vi "optionsAcq_readError.vi"(0 "option default":u16, 2 "option return":i32, 5 "error in (no error)":errorcluster, 9 "error ignore":bool) -> (15 "status":string, 16 "option":u16, 19 "error out":errorcluster)   [LabVIEW 2010, in "OSA.lvclass"]
doc: "SubVI to a <B>Thorlabs_OSA_64</B> object.\n\n[GOOP 1.0]"
uses:
  OSA.lvclass
  OSA20X_misc.lvlib
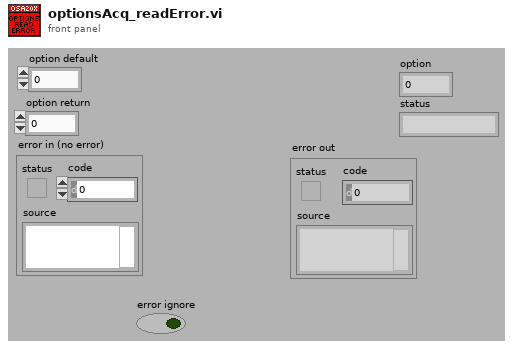
[diagram p1: front panel]
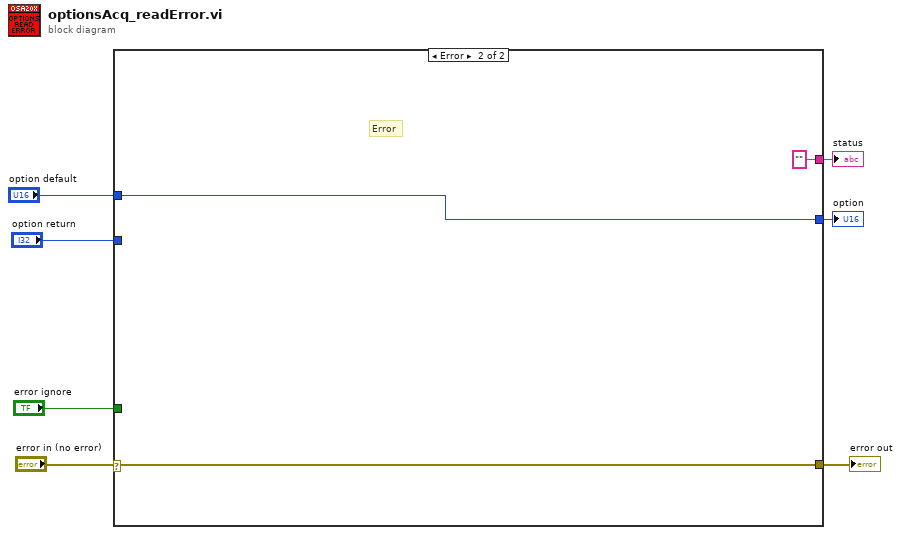
[diagram p0: block diagram]
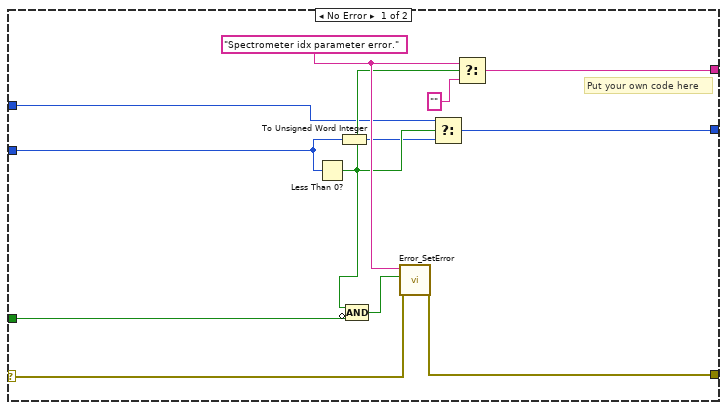
[diagram p2: hidden frame]
diagram:
  n1 = case shown="Error" "error in (no error)" {
    selector: "error in (no error)" -> [w9 w22]
    tunnel: [w8 w22] -> w7
    tunnel: "option return" -> [w14 _]
    tunnel: "option default" -> [w13 w21]
    tunnel: "error ignore" -> [w12 _]
    tunnel: [w11 w21] -> w2
    tunnel: [w10 ""] -> w1
    frame No Error {
      w18 = "Spectrometer idx parameter error." ("status")
      # "Put your own code here"
      n2 = Less Than 0?(x=w14) -> (x < 0?=w16:bool)
      n3 = To Unsigned Word Integer(number=w14) -> (unsigned 16bit integer=w15:u16)
      n4 = Compound Arithmetic op=AND(w16, invert w12) -> (w17:bool)
      n5 = call "Error_SetError.vi"("error in"=w9, "status (true)"=w17, "source(\"\")"=w18) -> ("error out"=w8:errorcluster)  [unwired: 4 in]
      n6 = Select(t=w13, s=w16, f=w15) -> (s? t:f=w11:u16)
      n7 = Select(t=w18, s=w16, f="") -> (s? t:f=w10:string)
    }
    frame Error {
      # "Error"
    }
  }
  "error out" <- w7
  "option" <- w2
  "status" <- w1
